vi "Single Trigger Pattern Truth.vi"(8 "error in":errorcluster, 10 "Pattern Truth":i32 caption="Pattern Mask" format="%.0b", 11 "Instrument Handle In":i32) -> (0 "error out":errorcluster, 3 "Instrument Handle Out":i32)   [LabVIEW 8.6, in "ZTScopeM.lvlib"]
doc: "Configure the trigger pattern truth."
uses:
  ZTScopeM.lvlib
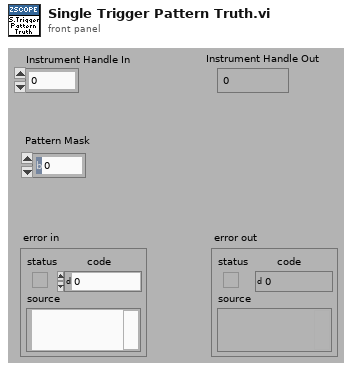
[diagram p1: front panel]
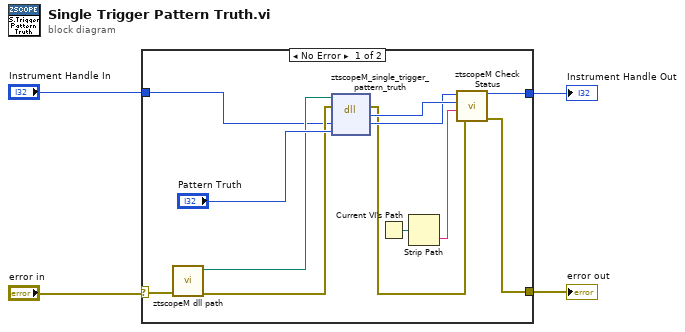
[diagram p0: block diagram]
diagram:
  n1 = case shown="No Error" "error in" {
    selector: "error in" -> [w9 w18]
    tunnel: [w11 w18] -> w3
    tunnel: [w12 w17] -> w2
    tunnel: "Instrument Handle In" -> [w5 w17]
    frame #0 {
      n2 = call "ztscopeM dll path.vi"("error in (no error)"=w9) -> ("error out"=w7:errorcluster, "<instrument>.dll path"=w8:path)  [unwired: 9 in]
      n3 = dll-call lib="C:/Program Files (x86)/National Instruments/LabVIEW 2013/instr.lib/ztscopem/ztscopeM.dll" fn="ztscopeM_single_trigger_pattern_truth"(path in=w8, error in=w7, "instrumentHandle"=w5, "patternTruth"="Pattern Truth") -> (error out=w6:errorcluster, w16:i32, "instrumentHandle"=w15:i32)  [unwired: 2 in, 1 out]
      n4 = Current VI's Path() -> (path=w14:path)
      n5 = Strip Path(path=w14) -> (name=w13:string)  [unwired: 1 out]
      n6 = call "ztscopeM Check Status.vi"("error in"=w6, "name of VI"=w13, "status (return code)"=w16, "instrument handle in"=w15) -> ("error out"=w11:errorcluster, "instrument handle out"=w12:i32)  [unwired: 2 out]
    }
    frame #1 {
    }
  }
  "Instrument Handle Out" <- w2
  "error out" <- w3
